vi "Example Secured TCP Client-Server.vi"() -> ()   [LabVIEW 2020]
uses:
  Connection.TCP-TLS.lvclass/Connection.TCP-TLS.ctl
  43a41480-018f-4496-923f-fa3aa5ba95d5.vi
  3dadd0ee-c965-4723-bd29-fb582b09aabd.vi
  dbc221b5-312b-4573-8364-df1029397b10.vi
  Read trusted entities.vi
  Write trusted entities.vi
  Connection.TCP-TLS.lvclass
  C:/Program Files (x86)/National Instruments/LabVIEW 2020/vi.lib/LabVIEW Open Source Project/Connection/Connection/Connection.lvclass
  <vilib>/LabVIEW Open Source Project/Connection/Connection/Connection.lvclass
panel:
  out "client certificate added":bool
  out "Auth Client?":bool
  out "server ready for TLS":bool
  out "client ready for TLS":bool
  out "server connected":bool
  out "client connected":bool
  out "Comm OK":bool
  out "value":dbl
  out "listener error":errorcluster
  out "client session error":errorcluster
  out "server session error":errorcluster
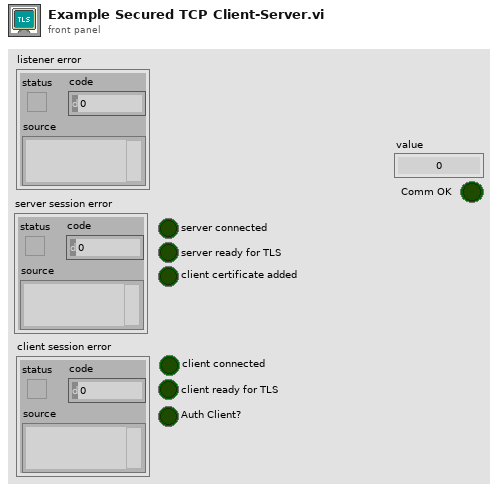
[diagram p1: front panel]
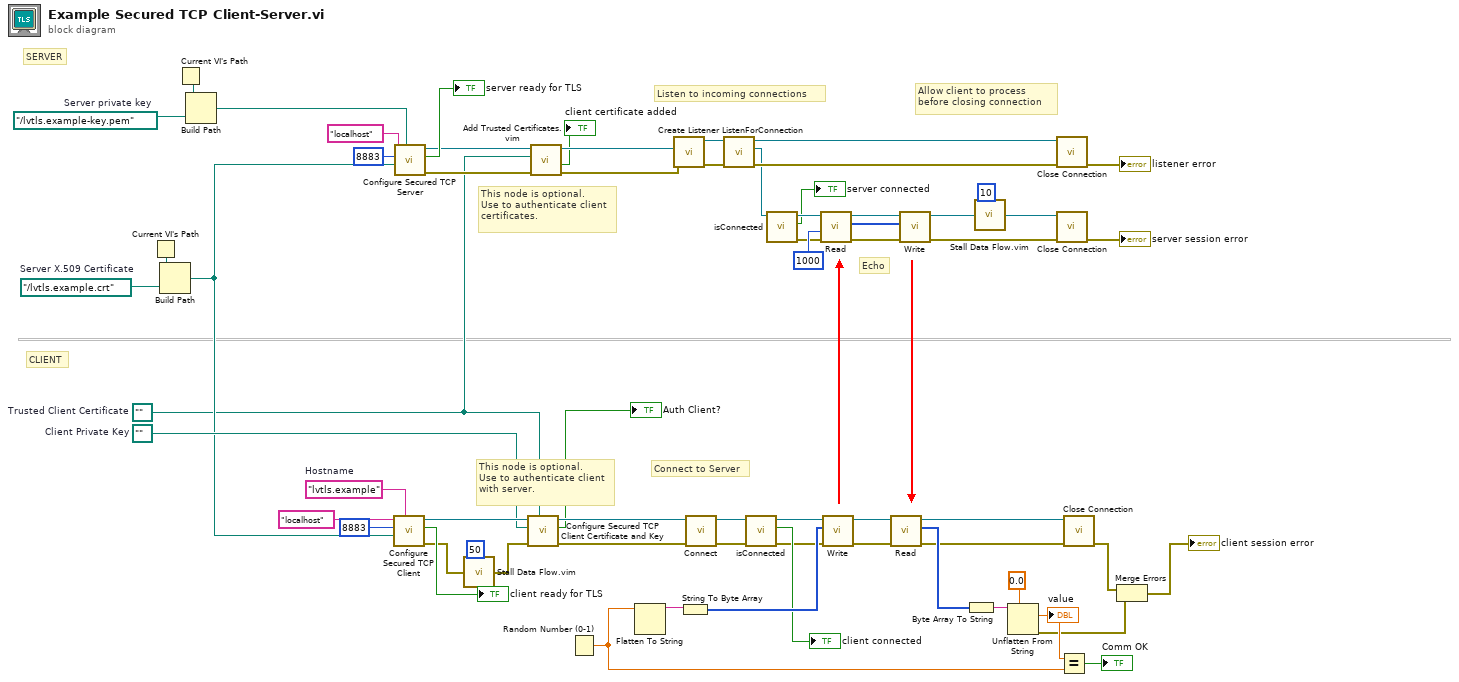
[diagram p0: block diagram]
diagram:
  w7 = path "../lvtls.example.crt"  # Server X.509 Certificate
  w1 = path ""  # Trusted Client Certificate
  w20 = path "../lvtls.example-key.pem"  # Server private key
  w37 = path ""  # Client Private Key
  w65 = "lvtls.example"  # Hostname
  # "This node is optional.\nUse to authenticate client\nwith server."
  # "This node is optional.\nUse to authenticate client\ncertificates."
  # "CLIENT"
  # "SERVER"
  # "Allow client to process\nbefore closing connection"
  # "Echo"
  # "Listen to incoming connections"
  # "Connect to Server"
  n1 = Current VI's Path() -> (path=w8:path)
  n2 = Build Path(base path=w8, name or relative path=w7) -> (appended path=w6:path)
  n3 = Current VI's Path() -> (path=w5:path)
  n4 = Build Path(base path=w5, name or relative path=w20) -> (appended path=w19:path)
  n5 = call "Configure Secured TCP Client.vi"("Hostname"=w65, "Server X.509 Certificate"=w6, "remote port (443)"=u16 8883 ("remote port (80)"), "address (localhost)"="localhost") -> ("error out"=w3:errorcluster, "Ready for SSL"=→"client ready for TLS":bool, "Secured TCP Connection"=w44:refnum<class "Connection.TCP-TLS.lvclass">)  [unwired: 5 in]
  n6 = call "Configure Secured TCP Server.vi"("Server private key"=w19, "Server X.509 Certificate"=w6, "remote port (443)"=u16 8883 ("remote port (80)"), "address (localhost)"="localhost") -> ("error out"=w11:errorcluster, "Ready for SSL"=→"server ready for TLS":bool, "Secured TCP Connection"=w12:refnum<class "Connection.TCP-TLS.lvclass">)  [unwired: 5 in]
  n7 = call "Stall Data Flow.vim"("value in"=w3, "milliseconds to wait"=u32 50) -> ("value out"=w2:errorcluster)  [unwired: 1 out]
  n8 = call "Configure Secured TCP Client Certificate and Key.vi"("Client X.509 Certificate"=w1, "error in (no error)"=w2, "Client Private Key"=w37, "Connection.TCP-TLS in"=w44) -> ("error out"=w42:errorcluster, "Auth Client?"=→"Auth Client?":bool, "Connection.TCP-TLS out"=w43:refnum<class "Connection.TCP-TLS.lvclass">)  [unwired: 5 in]
  n9 = call "Add Trusted Certificates.vim"("error in (no error)"=w11, "Trusted Certificate"=w1, "Connection.TCP-TLS in"=w12) -> ("error out"=w10:errorcluster, "certificate added"=→"client certificate added":bool, "Connection.TCP-TLS out"=w13:refnum<class "Connection.TCP-TLS.lvclass">)  [unwired: 6 in]
  n10 = Random Number (0-1)() -> (number: 0 to 1=w54:dbl)
  n11 = Flatten To String(anything=w54) -> (data string=w62:string)  [unwired: 3 in, 2 out]
  n12 = call <vilib>:"Create Listener.vi"("error in (no error)"=w10, "Connection Configuration"=w13) -> ("error out"=w32:errorcluster, "Listener"=w34:refnum<class "Connection.TCP-TLS.lvclass">)  [unwired: 8 in]
  n13 = String To Byte Array(string=w62) -> (unsigned byte array=w61:u8[])
  n14 = call <vilib>:"Connect.vi"("error in (no error)"=w42, "Connection in"=w43) -> ("error out"=w51:errorcluster, "Connection out"=w49:refnum<class "Connection.TCP-TLS.lvclass">)  [unwired: 8 in]
  n15 = call <vilib>:"ListenForConnection.vi"("error in (no error)"=w32, "Listener"=w34) -> ("error out"=w26:errorcluster, "Connection"=w24:refnum<class "Connection.lvclass">, "Listener out"=w33:refnum<class "Connection.TCP-TLS.lvclass">)  [unwired: 6 in, 1 out]
  n16 = call <vilib>:"isConnected.vi"("error in (no error)"=w51, "Connection in"=w49) -> ("error out"=w50:errorcluster, "connected"=→"client connected":bool, "Connection out"=w48:refnum<class "Connection.TCP-TLS.lvclass">)  [unwired: 7 in]
  n17 = call <vilib>:"isConnected.vi"("Connection in"=w24) -> ("error out"=w22:errorcluster, "connected"=→"server connected":bool, "Connection out"=w23:refnum<class "Connection.lvclass">)  [unwired: 8 in]
  n18 = call <vilib>:"Read.vi"("error in (no error)"=w22, "timeout (2000 ms)"=1000 ("bytes to read (100)"), "TCPConnection in"=w23) -> ("error out"=w28:errorcluster, "Bytes"=w29:u8[], "TCPConnection out"=w30:refnum<class "Connection.lvclass">)  [unwired: 4 in, 2 out]
  n19 = call <vilib>:"Write.vi"("error in (no error)"=w50, "Bytes"=w61, "Connection in"=w48) -> ("error out"=w63:errorcluster, "Connection"=w64:refnum<class "Connection.TCP-TLS.lvclass">)  [unwired: 7 in]
  n20 = call <vilib>:"Read.vi"("error in (no error)"=w63, "TCPConnection in"=w64) -> ("error out"=w57:errorcluster, "Bytes"=w60:u8[], "TCPConnection out"=w56:refnum<class "Connection.TCP-TLS.lvclass">)  [unwired: 5 in, 2 out]
  n21 = call <vilib>:"Write.vi"("error in (no error)"=w28, "Bytes"=w29, "Connection in"=w30) -> ("error out"=w15:errorcluster, "Connection"=w18:refnum<class "Connection.lvclass">)  [unwired: 7 in]
  n22 = Byte Array To String(unsigned byte array=w60) -> (string=w59:string)
  n23 = call "Stall Data Flow.vim"("value in"=w18, "milliseconds to wait"=u32 10) -> ("value out"=w17:refnum<class "Connection.lvclass">)  [unwired: 1 out]
  n24 = Unflatten From String(type=0.0, binary string=w59) -> (value=w55:dbl, error out=w47:errorcluster)  [unwired: 3 in, 1 out]
  "value" <- w55
  n25 = call <vilib>:"Close Connection.vi"("error in (no error)"=w26, "Connection in"=w33) -> ("error out"=→"listener error":errorcluster)  [unwired: 8 in, 1 out]
  n26 = call <vilib>:"Close Connection.vi"("error in (no error)"=w15, "Connection in"=w17) -> ("error out"=→"server session error":errorcluster)  [unwired: 8 in, 1 out]
  n27 = Equal?(x=w55, y=w54) -> (x = y?=→"Comm OK":bool)
  n28 = call <vilib>:"Close Connection.vi"("error in (no error)"=w57, "Connection in"=w56) -> ("error out"=w46:errorcluster)  [unwired: 8 in, 1 out]
  n29 = Merge Errors(w46, w47) -> (→"client session error":errorcluster)
